vi "RF_SetIQCaptureStart.vi"(7 "RFIndex":u32, 8 "error in (no error)":errorcluster) -> (0 "error out":errorcluster, 3 "return":i32)   [LabVIEW 2018]
uses:
  Common/Driver/rd.dll
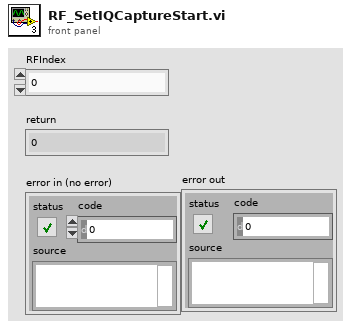
[diagram p1: front panel]
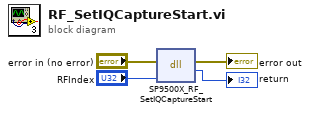
[diagram p0: block diagram]
diagram:
  n1 = dll-call lib="C:/rd/LabVIEW/Common/Driver/rd.dll" fn="SP9500X_RF_SetIQCaptureStart"(error in="error in (no error)", "RFIndex"="RFIndex") -> (error out=→"error out":errorcluster, "return"=→"return":i32)  [unwired: 3 in, 1 out]
